vi "Auton-SetDown.vi"(8 "error in (no error)":errorcluster, 10 "OnTopOf":dbl, 11 "Auton Event Queue Data":refnum<queue>) -> (0 "error out":errorcluster, 2 "Done":bool, 3 "Auton Event Queue Data 2":refnum<queue>)   [LabVIEW 2014]
uses:
  Robot Global Data.vi
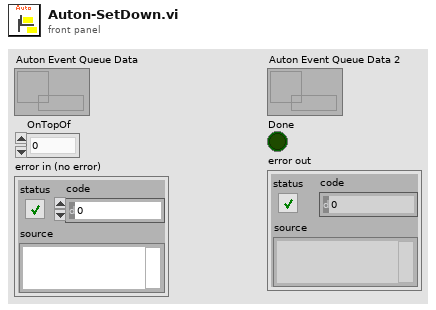
[diagram p1: front panel]
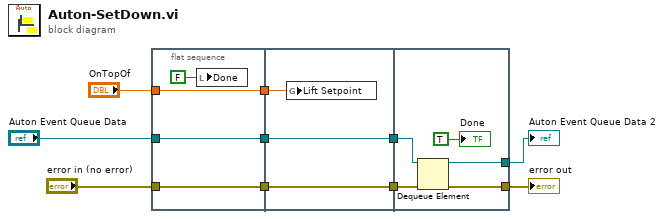
[diagram p0: block diagram]
diagram:
  n1 = flat-sequence {
    tunnel: "OnTopOf" -> [w14]
    tunnel: [w14] -> w9
    tunnel: "Auton Event Queue Data" -> [w12]
    tunnel: "error in (no error)" -> [w11]
    tunnel: [w12] -> w6
    tunnel: [w11] -> w5
    tunnel: w9 -> [w17]
    tunnel: w6 -> [w15]
    tunnel: w5 -> [w16]
    tunnel: [w16] -> w4
    tunnel: [w15] -> w3
    tunnel: w4 -> [w20]
    tunnel: w3 -> [w21]
    tunnel: [w19] -> w2
    tunnel: [w18] -> w1
    frame #0 {
      n2 = local write "Done"(FALSE ("Done")) -> ()
    }
    frame #1 {
      n3 = global write "Robot Global Data.vi" "Lift Setpoint"(w17) -> ()
    }
    frame #2 {
      n4 = Dequeue Element(queue=w21, error in (no error)=w20) -> (queue out=w18:refnum<queue>, error out=w19:errorcluster)  [unwired: 1 in, 2 out]
      "Done" <- TRUE
    }
  }
  "Auton Event Queue Data 2" <- w1
  "error out" <- w2
